vi "Wait For Acquisition Complete.vi"(8 "error in (no error)":errorcluster, 10 "Maximum Time (10000ms)":u32=10000, 11 "VISA resource name":refnum<visa-resource-name>) -> (0 "error out":errorcluster, 3 "VISA resource name out":refnum<visa-resource-name>)   [LabVIEW 2012, in "Agilent 8000 Series.lvlib"]
doc: "Waits for the instrument to complete the execution of all pending operations. The <B>Timeout</B> control specifies the maximum time to wait for operation complete in milliseconds."
uses:
  Agilent 8000 Series.lvlib
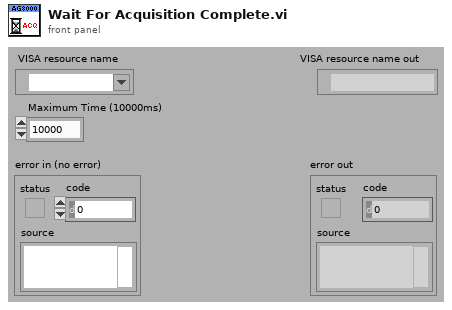
[diagram p1: front panel]
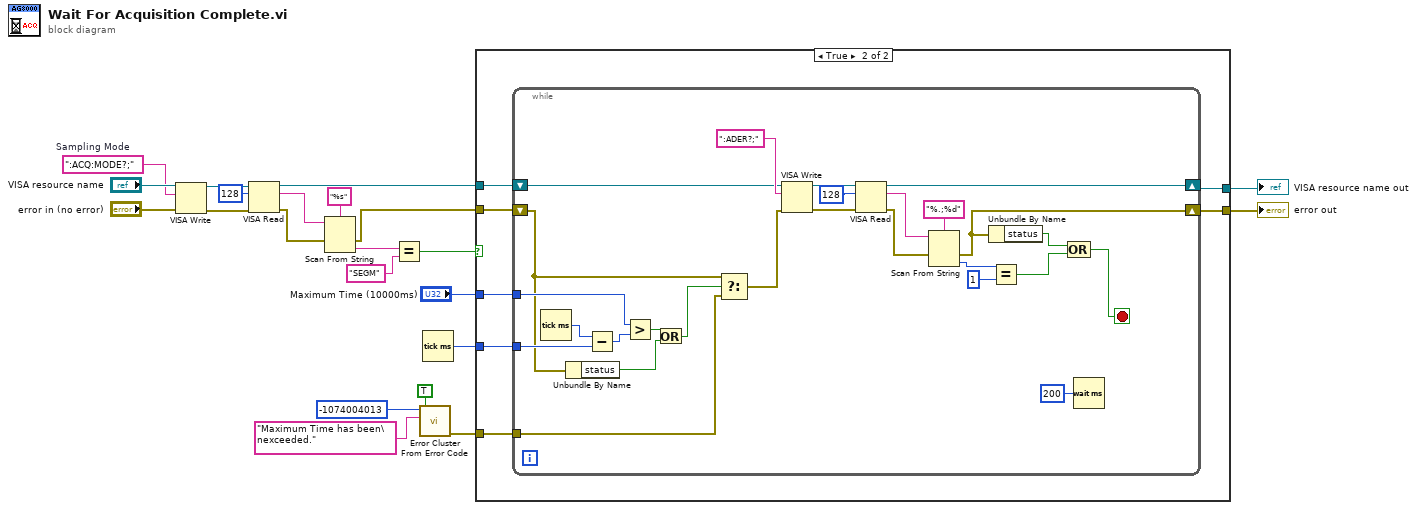
[diagram p0: block diagram]
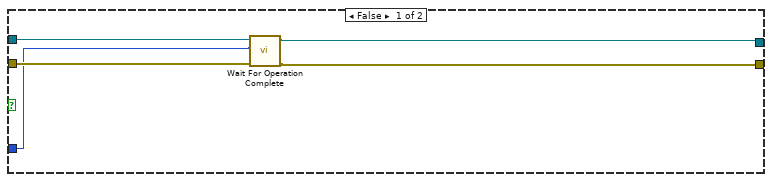
[diagram p2: hidden frame]
diagram:
  w18 = ":ACQ:MODE?;"  # Sampling Mode
  n1 = VISA Write(VISA resource name="VISA resource name", write buffer=w18, error in (no error)="error in (no error)") -> (VISA resource name out=w19:refnum<visa-resource-name>, error out=w20:errorcluster)  [unwired: 1 out]
  n2 = VISA Read(VISA resource name=w19, byte count=u32 128, error in (no error)=w20) -> (VISA resource name out=w12:refnum<visa-resource-name>, read buffer=w7:string, error out=w11:errorcluster)  [unwired: 1 out]
  n3 = Scan From String(format string="%s", input string=w7, error in=w11) -> (error out=w10:errorcluster, output 1=w9:string)  [unwired: 2 in, 2 out]
  n4 = Equal?(x=w9, y="SEGM") -> (x = y?=w14:bool)
  n5 = call <vilib>:"Error Cluster From Error Code.vi"("show call chain? (False)"=TRUE, "error message (\"\")"="Maximum Time has been\nexceeded." ("error message (\"\")"), "error code (0)"=-1074004013) -> ("error out"=w1:errorcluster)  [unwired: 6 in]
  n6 = Tick Count (ms)() -> (millisecond timer value=w6:u32)
  n7 = case shown="True" w14 {
    tunnel: w12 -> [w23 w34]
    tunnel: w10 -> [w25 w33]
    tunnel: [w27 w32] -> w16
    tunnel: [w26 w31] -> w15
    tunnel: w6 -> [_ w30]
    tunnel: "Maximum Time (10000ms)" -> [w24 w29]
    tunnel: w1 -> [_ w28]
    frame False {
      n8 = call "Wait For Operation Complete.vi"("error in (no error)"=w25, "Maximum Time (10000ms)"=w24, "VISA resource name"=w23) -> ("error out"=w26:errorcluster, "VISA resource name out"=w27:refnum<visa-resource-name>)  [unwired: 7 in]
    }
    frame True {
      n9 = while {
        shift-right: [w49] -> w31
        shift-left: w33 -> [w39]
        shift-right: [w51] -> w32
        shift-left: w34 -> [w59]
        tunnel: w30 -> [w43]
        tunnel: w29 -> [w41]
        tunnel: w28 -> [w37]
        stop <- w52 stop-if-true
        n10 = Tick Count (ms)() -> (millisecond timer value=w44:u32)
        n11 = Unbundle By Name(w39) -> ("status"=w35:bool)
        n12 = Subtract(x=w44, y=w43) -> (x-y=w42:u32)
        n13 = Greater?(x=w41, y=w42) -> (0:w40:bool)
        n14 = Or(x=w40, y=w35) -> (x .or. y?=w38:bool)
        n15 = Select(t=w39, s=w38, f=w37) -> (s? t:f=w36:errorcluster)
        n16 = VISA Write(VISA resource name=w59, write buffer=":ADER?;", error in (no error)=w36) -> (VISA resource name out=w58:refnum<visa-resource-name>, error out=w57:errorcluster)  [unwired: 1 out]
        n17 = VISA Read(VISA resource name=w58, byte count=u32 128, error in (no error)=w57) -> (VISA resource name out=w51:refnum<visa-resource-name>, read buffer=w48:string, error out=w45:errorcluster)  [unwired: 1 out]
        n18 = Scan From String(format string="%.;%d", input string=w48, error in=w45) -> (error out=w49:errorcluster, output 1=w46:i32)  [unwired: 2 in, 2 out]
        n19 = Unbundle By Name(w49) -> ("status"=w54:bool)
        n20 = Equal?(x=w46, y=1) -> (x = y?=w53:bool)
        n21 = Compound Arithmetic op=OR(w54, w53) -> (w52:bool)
        n22 = Wait (ms)(milliseconds to wait=u32 200) -> ()  [unwired: 1 out]
      }
    }
  }
  "error out" <- w15
  "VISA resource name out" <- w16
